vi "USB-TC_Buffer_Dbl_VIG.vi"(7 "Operation":enum16{"get data", "set data", "initialize"}(ring)=enum."set data", 8 "error in":errorcluster, 11 "Numeric":dbl) -> (0 "error out":errorcluster, 3 "Numeric":dbl)   [LabVIEW 2010]
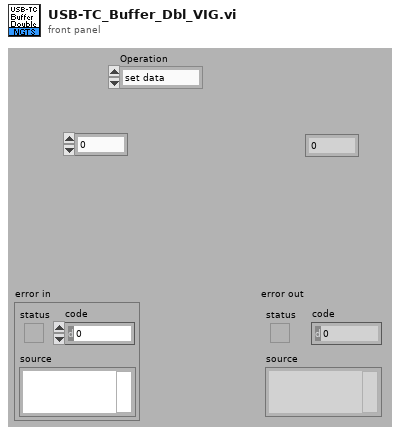
[diagram p1: front panel]
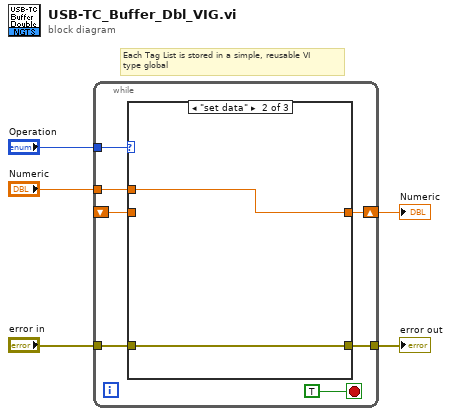
[diagram p0: block diagram]
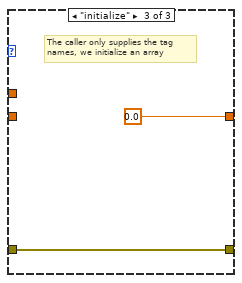
[diagram p3: hidden frame]
diagram:
  # "Each Tag List is stored in a simple, reusable VI\ntype global"
  n1 = while {
    tunnel: "Operation" -> [w12]
    shift-right: [w10] -> w3
    shift-left: _ -> [w8]
    tunnel: "Numeric" -> [w9]
    tunnel: "error in" -> [w7]
    tunnel: [w6] -> w1
    stop <- TRUE stop-if-true
    n2 = case shown="\"set data\"" w12 {
      tunnel: [w14 w16 0.0 ("element")] -> w10
      tunnel: w9 -> [_ w16 _]
      tunnel: w8 -> [w14 _ _]
      tunnel: w7 -> [w13 w15 w18]
      tunnel: [w13 w15 w18] -> w6
      frame "get data", Default {
      }
      frame "set data" {
      }
      frame "initialize" {
        # "The caller only supplies the tag\nnames, we initialize an array"
      }
    }
  }
  "error out" <- w1
  "Numeric" <- w3
